vi "Get Start.vi"(8 "error in (no error)":errorcluster, 11 "Map in":refnum<class "Maze.lvclass">) -> (0 "error out":errorcluster, 2 "Start Vectors":T1, 3 "Map out":refnum<class "Maze.lvclass">)   [LabVIEW 2021, in "Maze.lvclass"]
uses:
  Maze.lvclass
  Position.ctl
  Maze.lvclass/Maze.ctl
panel:
  out "Row":u64
  out "Col":u64
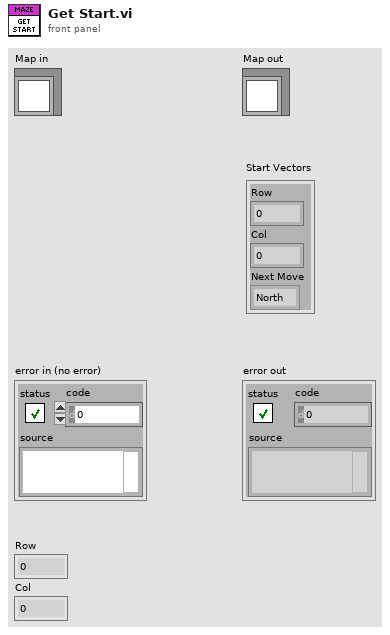
[diagram p1: front panel]
types:
  T1 = typedef "Maze.lvclass/Position.ctl" = cluster{"Row":u64, "Col":u64, "Next Move":enum16{"North", "East", "South", "West", "Halt"}}
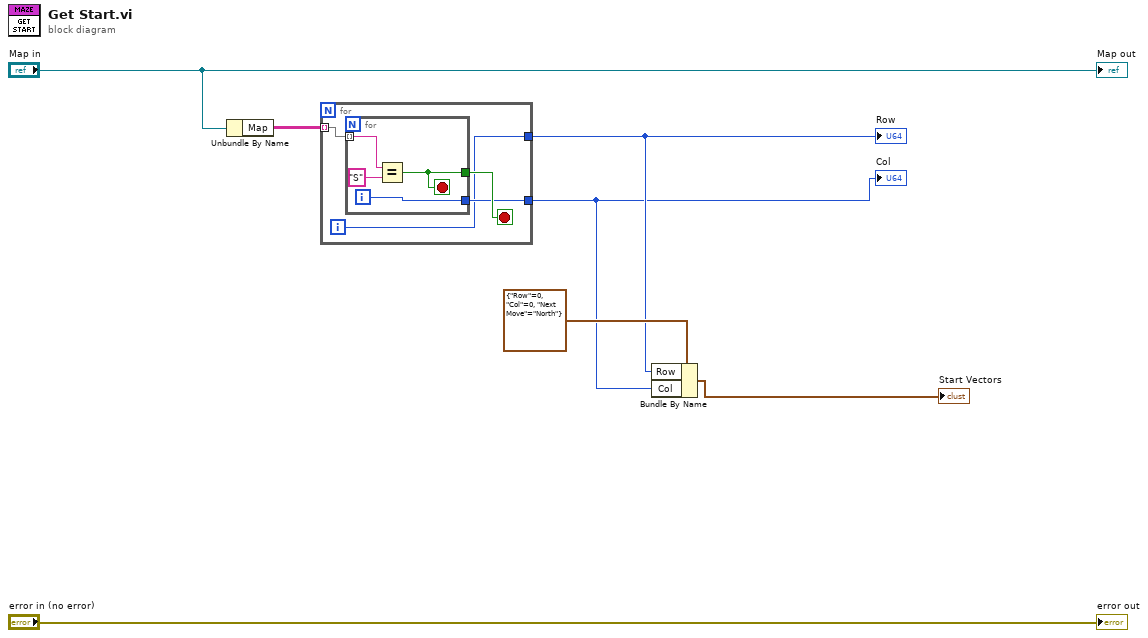
[diagram p0: block diagram]
diagram:
  n1 = Unbundle By Name("Map in") -> ("Map"=w5:string[][])
  n2 = for {
    tunnel: w5 -> [w11] mode=indexing
    tunnel: [w9] -> w2
    tunnel: [w8] -> w3
    i -> [w8]
    stop <- w10 stop-if-true
    n3 = for {
      tunnel: w11 -> [w15] mode=indexing
      tunnel: [w13] -> w10
      tunnel: [w12] -> w9
      i -> [w12]
      stop <- w13 stop-if-true
      n4 = Equal?(x=w15, y="S") -> (x = y?=w13:bool)
    }
  }
  "Col" <- w2
  "Row" <- w3
  n5 = Bundle By Name(cluster=T1 {"Row"=0, "Col"=0, "Next Move"=enum."North"} ("Cluster"), "Row"=w3, "Col"=w2) -> (→"Start Vectors":T1)
  "error out" <- "error in (no error)"
  "Map out" <- "Map in"
